vi "Calculate I2C Wave.vi"(8 "error in (no error)":errorcluster, 11 "Devices in":refnum<class "Devices.lvclass">) -> (0 "error out":errorcluster, 3 "Devices out":refnum<class "Devices.lvclass">)   [LabVIEW 2020, in "Devices.lvclass"]
uses:
  Devices.lvclass
  Devices.lvclass/Devices.ctl
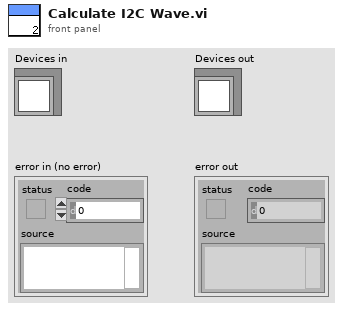
[diagram p1: front panel]
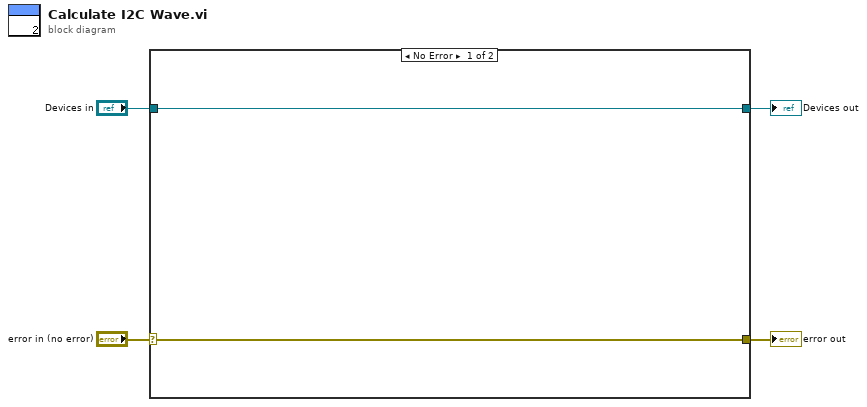
[diagram p0: block diagram]
diagram:
  n1 = case shown="No Error" "error in (no error)" {
    selector: "error in (no error)" -> [w6 w8]
    tunnel: [w6 w8] -> w3
    tunnel: [w5 w7] -> w1
    tunnel: "Devices in" -> [w5 w7]
    frame No Error {
    }
    frame Error {
    }
  }
  "error out" <- w3
  "Devices out" <- w1
